vi "Close Connection.vi"(8 "error in (no error)":errorcluster, 11 "GenNet Variant Protocol in":refnum<class "GenNet Variant Protocol.lvclass">) -> (0 "error out":errorcluster, 3 "GenNet Variant Protocol out":refnum<class "GenNet Variant Protocol.lvclass">)   [LabVIEW 2022 SP3, in "hse-gennet.lvlib" / "GenNet Variant Protocol.lvclass"]
doc: "____\nHAMPEL SOFTWARE ENGINEERING v3.8.0 (2023-12-18 14:41)"
uses:
  GenNet Variant Protocol.lvclass
  GenNet Protocol.lvclass
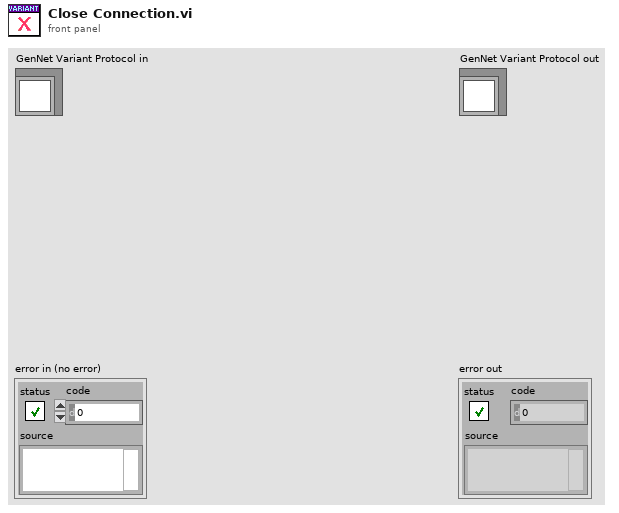
[diagram p1: front panel]
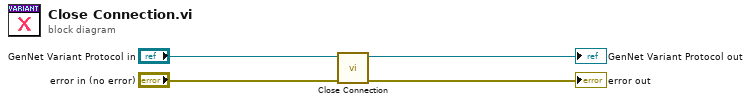
[diagram p0: block diagram]
diagram:
  n1 = call-parent "Close Connection.vi"("error in (no error)"="error in (no error)", "GenNet Protocol in"="GenNet Variant Protocol in") -> ("error out"=→"error out":errorcluster, "GenNet Protocol out"=→"GenNet Variant Protocol out":refnum<class "GenNet Variant Protocol.lvclass">)  [unwired: 8 in]
